vi "cluster_to_ini_file.vi"(8 "error in (no error)":errorcluster, 10 "data":variant, 11 "iniFilePath":path) -> (0 "error out":errorcluster)   [LabVIEW 2015, in "ini_work_Library.lvlib"]
doc: "Write any cluster to specified ini file\n\nCreated by Artem Shevelev\nshevelev.pro\nartem@shevelev.pro\nLabVIEW Portal: https://labviewportal.org/memberlist.php?mode=viewprofile&u=2340"
uses:
  ini_work_Library.lvlib
  <vilib>/Utility/config.llb/NI_LVConfig.lvlib
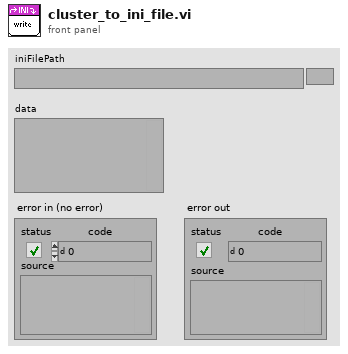
[diagram p1: front panel]
types:
  T1 = typedef "NI_LVConfig.lvlib/Config Data RefNum.ctl" = refnum<k1>
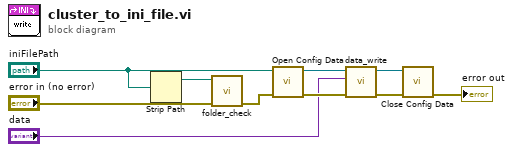
[diagram p0: block diagram]
diagram:
  n1 = Strip Path(path="iniFilePath") -> (stripped path=w4:path)  [unwired: 1 out]
  n2 = call "folder_check.vi"("error in (no error)"="error in (no error)", "stripped path"=w4) -> ("error out"=w1:errorcluster)  [unwired: 9 in]
  n3 = call <vilib>:"Open Config Data.vi"("error in (no error)"=w1, "configuration file path"="iniFilePath") -> ("error out"=w7:errorcluster, "refnum"=w10:T1)  [unwired: 7 in, 1 out]
  n4 = call "data_write.vi"("error in (no error)"=w7, "data"="data", "ini_file_refnum"=w10) -> ("error out"=w8:errorcluster, "ini_file_refnum_out"=w9:T1)  [unwired: 7 in]
  n5 = call <vilib>:"Close Config Data.vi"("error in (no error)"=w8, "refnum"=w9) -> ("error out"=→"error out":errorcluster)  [unwired: 8 in, 1 out]
